vi "Text File Read Display.vi"() -> ()   [LabVIEW 2014]
panel:
  out "dt":dbl
  out "size(s)":i32
  out "n pts":dbl
  in  "Exit Button":bool
  in  "Decimator":i32=1 min=1
  in  "Upload Button":bool
  out "Waveform Graph":waveform(dbl)(graph)
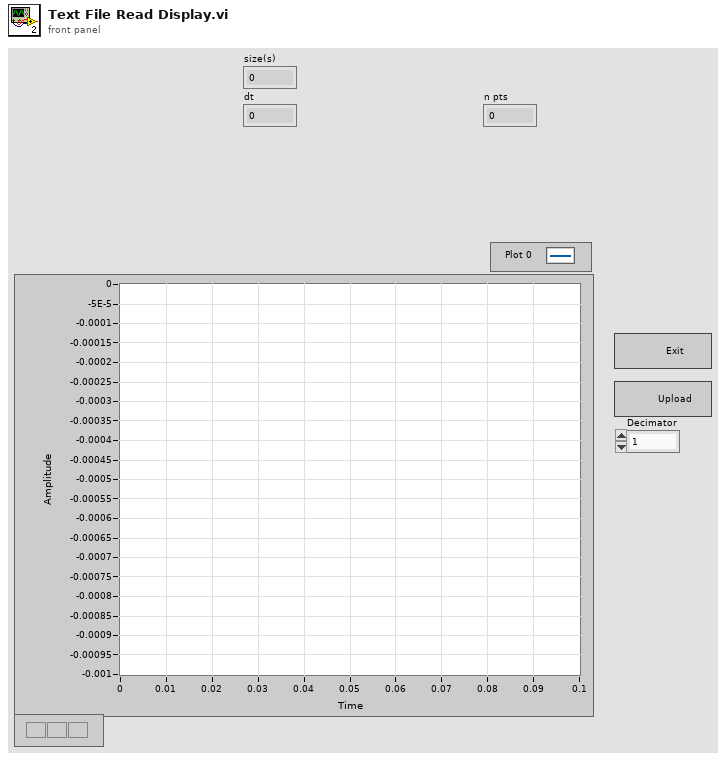
[diagram p1: front panel]
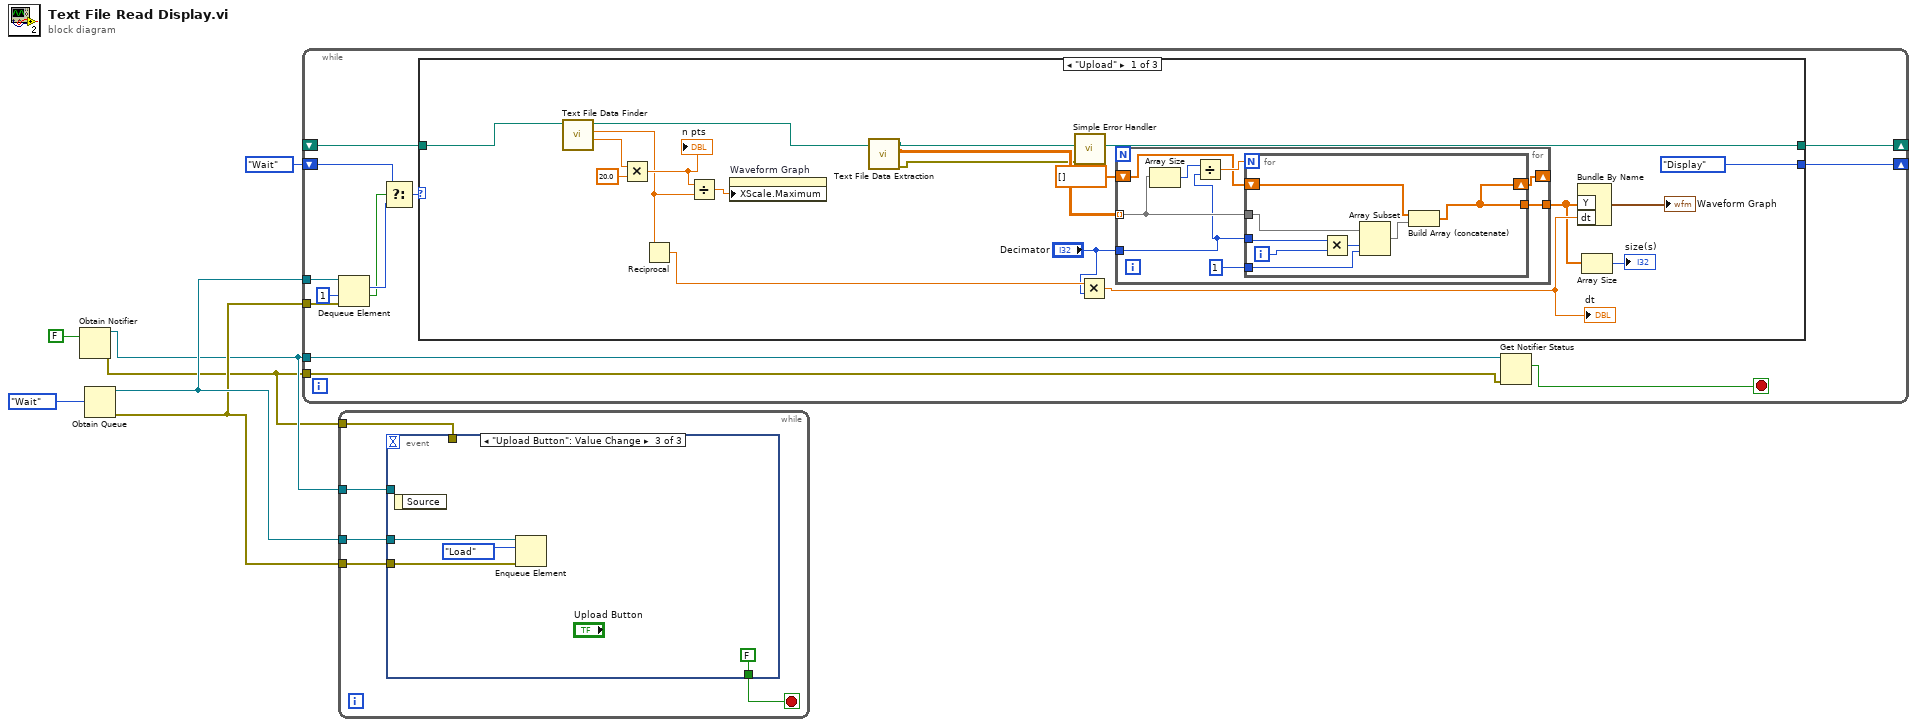
[diagram p0: block diagram]
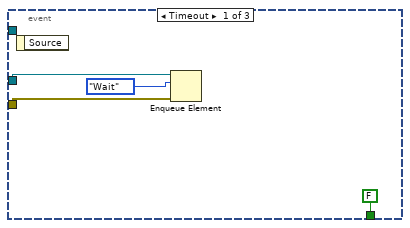
[diagram p2: hidden frame]
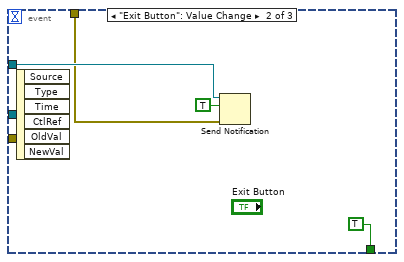
[diagram p3: hidden frame]
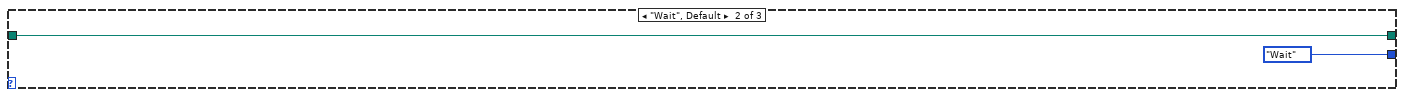
[diagram p4: hidden frame]
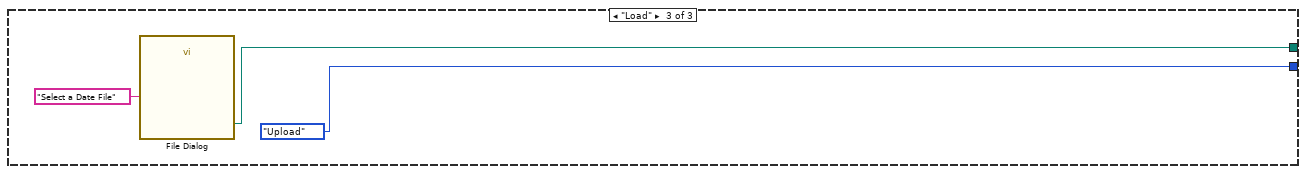
[diagram p5: hidden frame]
diagram:
  n1 = Obtain Notifier(notification data type=FALSE) -> (notifier out=w3:refnum<notifier>, error out=w2:errorcluster)  [unwired: 3 in, 1 out]
  n2 = Obtain Queue(element data type=enum16{"Upload", "Load", "Display", "Wait"}."Wait") -> (queue out=w7:refnum<queue>, error out=w5:errorcluster)  [unwired: 4 in, 1 out]
  n3 = while {
    tunnel: w7 -> [w20]
    tunnel: w5 -> [w19]
    shift-right: [w18] -> _
    shift-left: _ -> [w11]
    shift-right: [w12] -> _
    shift-left: enum16{"Upload", "Load", "Display", "Wait"}."Wait" -> [w13]
    tunnel: w3 -> [w10]
    tunnel: w2 -> [w9]
    stop <- w8 stop-if-true
    n4 = Dequeue Element(queue=w20, timeout in ms (-1)=1, error in (no error)=w19) -> (element=w16:enum16{"Upload", "Load", "Display", "Wait"}, timed out?=w14:bool)  [unwired: 2 out]
    n5 = Select(t=w13, s=w14, f=w16) -> (s? t:f=w15:enum16{"Upload", "Load", "Display", "Wait"})
    n6 = case shown="\"Upload\"" w15 {
      tunnel: [w24 w56 w58] -> w18
      tunnel: [enum16{"Upload", "Load", "Display", "Wait"}."Display" enum16{"Upload", "Load", "Display", "Wait"}."Wait" enum16{"Upload", "Load", "Display", "Wait"}."Upload"] -> w12
      tunnel: w11 -> [w38 w56 _]
      frame "Upload" {
        n7 = call "Text File Data Finder.vi"("File Path Control"=w38) -> ("Total Amount of Points"=w36:dbl, "Sample Rate"=w31:dbl, "File Path Indicator"=w25:path)  [unwired: 8 in]
        n8 = Multiply(x=w36, y=20.0) -> (x*y=w32:dbl)
        "n pts" <- w32
        n9 = Reciprocal(x=w31) -> (1/x=w34:dbl)
        n10 = Divide(x=w32, y=w31) -> (x/y=w30:dbl)
        n11 = property on="Waveform Graph" class="WFGraph (strict)"("XScale.Maximum"=w30) -> ()  [unwired: 2 in, 2 out]
        n12 = call "Text File Data Extraction.vi"("File Path Input"=w25) -> ("error out"=w22:errorcluster, "Array"=w23:dbl[][], "File Path Output"=w24:path)  [unwired: 8 in]
        n13 = call <vilib>:"Simple Error Handler.vi"("error in (no error)"=w22) -> ()  [unwired: 4 in, 5 out]
        n14 = Multiply(x=w34, y="Decimator") -> (x*y=w33:dbl)
        "dt" <- w33
        n15 = for {
          tunnel: [w46] -> w27
          tunnel: w23 -> [w44] mode=indexing
          tunnel: "Decimator" -> [w41]
          shift-right: [w40] -> _
          shift-left: dbl[] [] -> [w39]
          n16 = Array Size(array=w44) -> (size(s)=w43:i32)
          n17 = Divide(x=w43, y=w41) -> (x/y=w42:dbl)
          n18 = for {
            N: w42 -> [_]
            tunnel: w41 -> [w47]
            tunnel: [w50] -> w46
            tunnel: w44 -> [w51]
            shift-right: [w50] -> w40
            shift-left: w39 -> [w52]
            tunnel: 1 ("y") -> [w49]
            i -> [w48]
            n19 = Multiply(x=w47, y=w48) -> (x*y=w54:i32)
            n20 = Array Subset(array=w51, index=w54, length=w49) -> (w53:dbl[])
            n21 = Build Array (concatenate)(w52, w53) -> (w50:dbl[])
          }
        }
        n22 = Bundle By Name("Y"=w27, "dt"=w33) -> (→"Waveform Graph":waveform(dbl))  [unwired: 1 in]
        n23 = Array Size(array=w27) -> (size(s)=→"size(s)":i32)
      }
      frame "Wait", Default {
      }
      frame "Load" {
        n24 = call "File Dialog"("prompt"="Select a Date File") -> ("selected path"=w58:path)  [unwired: 11 in, 3 out]
      }
    }
    n25 = Get Notifier Status(notifier=w10, error in (no error)=w9) -> (current notification=w8:bool)  [unwired: 4 out]
  }
  n26 = while {
    tunnel: w7 -> [w64]
    tunnel: w5 -> [w63]
    tunnel: w3 -> [w62]
    tunnel: w2 -> [w61]
    stop <- w60 stop-if-true
    n27 = event shown="[2] \"Upload Button\": Value Change" {
      selector: _ -> [_ _ _]
      dyn-events: _ -> [_ _ _]
      timeout: _ -> [_ _ _]
      tunnel: w64 -> [w68 _ w76]
      tunnel: w63 -> [w67 _ w75]
      tunnel: w62 -> [_ w72 _]
      tunnel: w61 -> [_ w71 _]
      tunnel: [FALSE ("notification") TRUE ("notification") FALSE ("notification")] -> w60
      event Timeout {
        n28 = event-data() -> ()  [unwired: 1 in, 1 out]
        n29 = Enqueue Element(queue=w68, element=enum16{"Upload", "Load", "Display", "Wait"}."Wait", error in (no error)=w67) -> ()  [unwired: 1 in, 3 out]
      }
      event "Exit Button": Value Change {
        n30 = event-data() -> ()  [unwired: 1 in, 6 out]
        n31 = Send Notification(notification=TRUE, notifier=w72, error in (no error)=w71) -> ()  [unwired: 2 out]
      }
      event "Upload Button": Value Change {
        n32 = event-data() -> ()  [unwired: 1 in, 1 out]
        n33 = Enqueue Element(queue=w76, element=enum16{"Upload", "Load", "Display", "Wait"}."Load", error in (no error)=w75) -> ()  [unwired: 1 in, 3 out]
      }
    }
  }
